vi "LVClass_HasoData ctor from copy.vi"(0 "HasoData (const)":refnum<class "HasoData.lvclass">, 5 "HasoData toCopy":refnum<class "HasoData.lvclass">, 11 "error in (no error)":errorcluster) -> (4 "HasoData (new)":refnum<class "HasoData.lvclass">, 6 "HasoData toCopy (dup)":refnum<class "HasoData.lvclass">, 15 "error out":errorcluster)   [LabVIEW 2020, in "HasoData.lvclass"]
doc: "HasoData constructor from copy.\n\n--------------------------------------------------------------------------------\n\n<B>HasoDataIn </B> : Constant Pointer to HasoData object.\n<B>HasoDataOut </B> : Constant Pointer to HasoData object.\n<B>HasoData_src </B> : HasoData object to copy.\n<B>ErrorIn </B> : Error\n<B>ErrorOut </B> : Error\n\n--------------------------------------------------------------------------------"
uses:
  HasoData.lvclass
  Controls/Handle creation.ctl
  HasoData.lvclass/HasoData.ctl
  LVClass_HasoData Read HasoData - property.vi
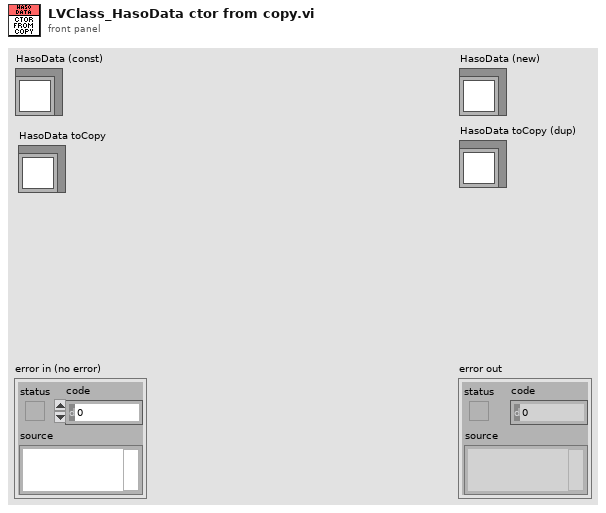
[diagram p1: front panel]
types:
  T1 = typedef "Handle creation.ctl" = enum16{"By ctor", "By write function"}
  T2 = typedef "ClassID.ctl" = i64
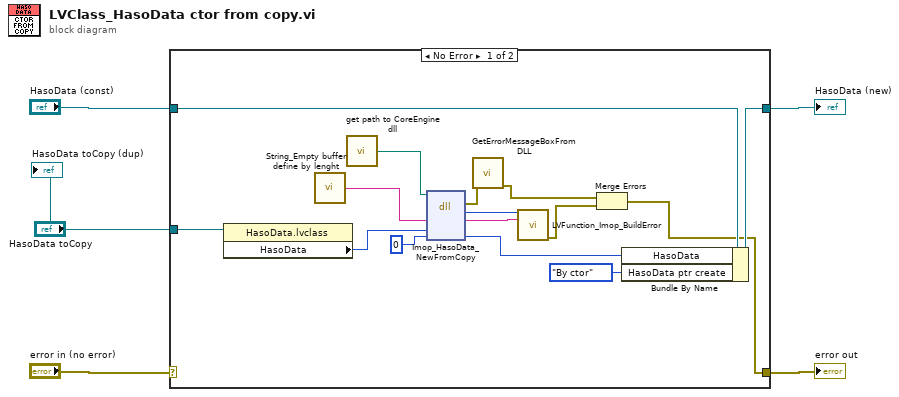
[diagram p0: block diagram]
diagram:
  n1 = case shown="No Error" "error in (no error)" {
    selector: "error in (no error)" -> [_ w22]
    tunnel: [w6 w22] -> w2
    tunnel: [w17 w21] -> w3
    tunnel: "HasoData (const)" -> [w18 w21]
    tunnel: "HasoData toCopy" -> [w11 _]
    frame No Error {
      n2 = property class="HasoData.lvclass"(reference=w11) -> ("HasoData"=w10:T2)  [unwired: 1 in, 2 out]
      n3 = call "String_Empty buffer define by lenght.vi"() -> ("Empty buffer"=w16:string)  [unwired: 1 in]
      n4 = call "get path to CoreEngine dll.vi"() -> ("path to wavekit library"=w15:path)  [unwired: 14 in, 1 out]
      n5 = dll-call lib="D:/soft/HASO_v3/SVN_trunk/ImOpCoreEngine4_LV2011/DLLs/c_interface_vc100.dll" fn="Imop_HasoData_NewFromCopy"(path in=w15, "message"=w16, "HasoDataToCopy"=w10, "HasoData"=0 ("objet")) -> (error out=w14:errorcluster, "return type"=w20:i32, "message"=w19:string, "HasoData"=w12:i64)  [unwired: 3 in, 1 out]
      n6 = call "GetErrorMessageBoxFromDLL.vi"("error IN"=w14) -> ("error OUT"=w8:errorcluster)  [unwired: 10 in]
      n7 = call "LVFunction_Imop_BuildError.vi"("code"=w20, "String to Prepend to source (\"\")"=w19) -> ("error out"=w7:errorcluster)  [unwired: 13 in]
      n8 = Merge Errors(w8, w7) -> (w6:errorcluster)
      n9 = Bundle By Name(cluster=w18, "HasoData"=w12, "HasoData ptr create"=Handle_creation."By ctor") -> (w17:refnum<class "HasoData.lvclass">)
    }
    frame Error {
    }
  }
  "error out" <- w2
  "HasoData (new)" <- w3
  "HasoData toCopy (dup)" <- "HasoData toCopy"
